vi "Smart baby safety and monitoring system.vi"() -> ()   [LabVIEW 2022 SP3]
uses:
  <vilib>/DAQmx/read.llb/DAQmx Read (Analog 1D DBL NChan 1Samp).vi
  <vilib>/DAQmx/write.llb/DAQmx Write (Digital Bool 1Line 1Point).vi
  <vilib>/DAQmx/create/channels.llb/DAQmx Create Channel (DO-Digital Output).vi
  <vilib>/DAQmx/create/channels.llb/DAQmx Create Channel (AI-Voltage-Basic).vi
  <vilib>/DAQmx/miscellaneous.llb/DAQmx Fill In Error Info.vi
panel:
  out "Cry Detected":bool
  in  "Fan Control":dbl
  in  "Vibration":tag
  out "Boolean":bool
  in  "Microphone":tag
  out "Microrphone":dbl(knob) scale=0.0..5000.0
  out "Microphone":dbl format="%0.2f"
  out "Vibration":dbl(knob) scale=-2.0..12.0
  out "Fan Speed":dbl
  out "Final":dbl
  out "Fan Activated":bool
  in  "Temp and Hum":tag
  out "Temperature":dbl(graph)
  out "Temperature":dbl(knob) scale=10.0..40.0
  out "Numeric":dbl
  out "Temperature":dbl
  out "Humidity":dbl(graph)
  out "Humidity":dbl
  out "Waveform Chart":T1(graph)
  out "Humidity":dbl(knob) scale=0.0..100.0
  in  "DAQmx Physical Channel":tag
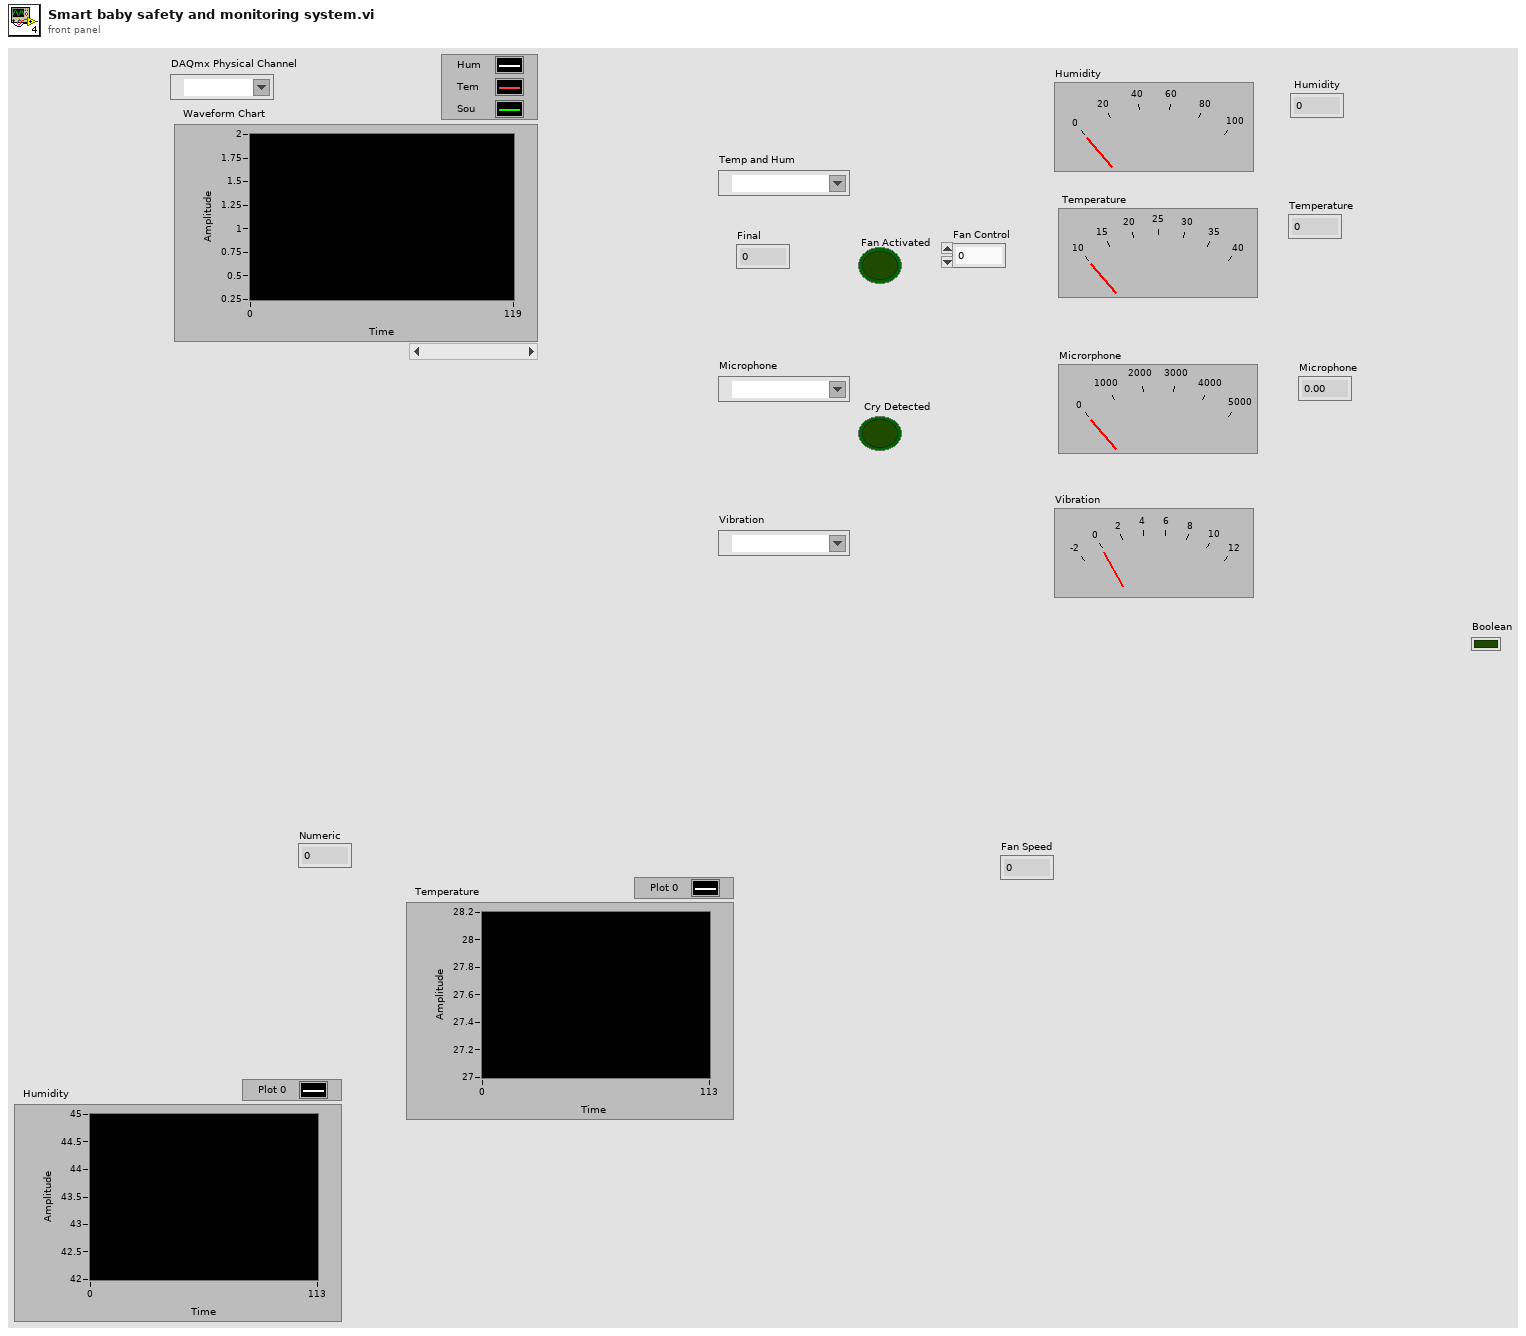
[diagram p1: front panel]
types:
  T1 = cluster{"Waveform":dbl, "Waveform":dbl, "Waveform":dbl}
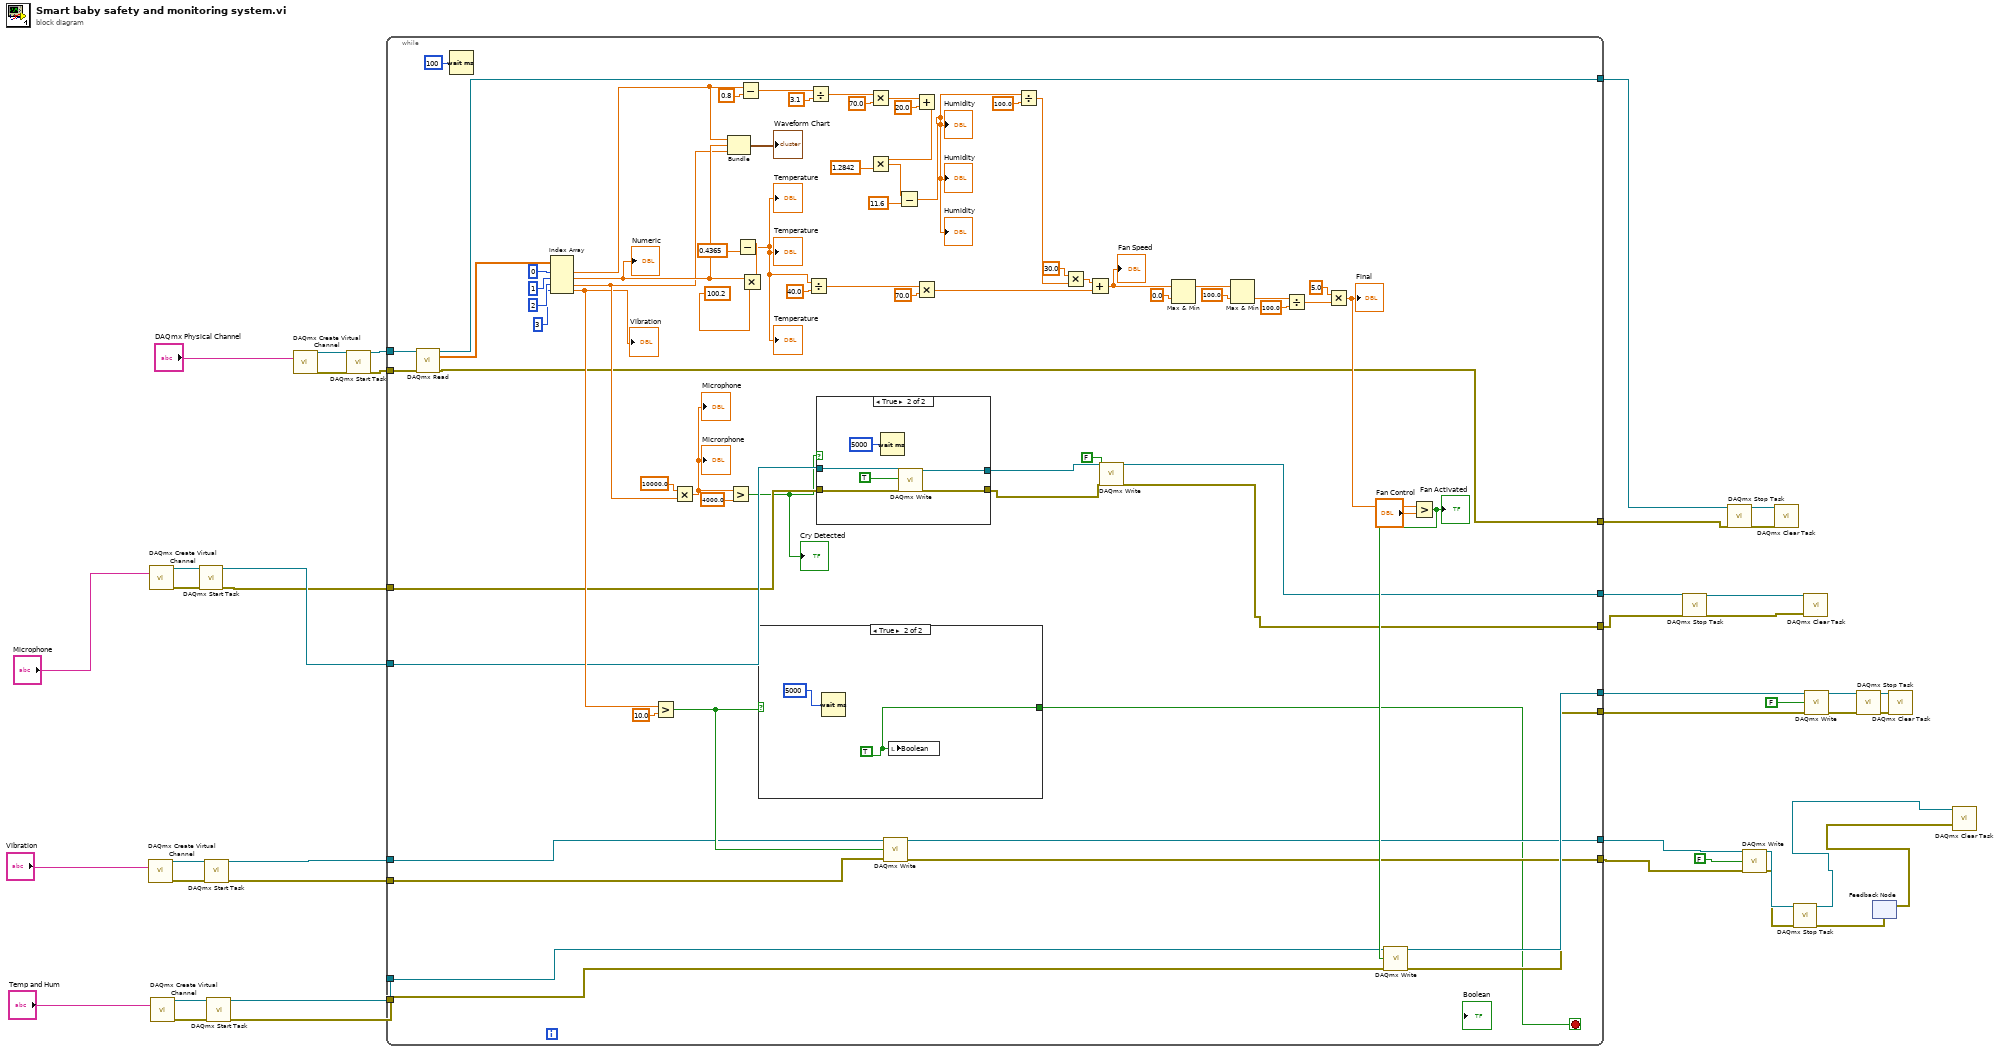
[diagram p0: block diagram]
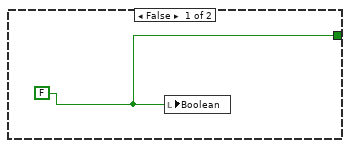
[diagram p2: hidden frame]
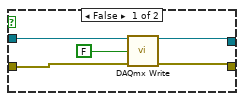
[diagram p3: hidden frame]
diagram:
  n1 = call-poly <vilib>:"DAQmx Create Virtual Channel.vi"("lines"="Vibration") -> ("task out"=w18:refnum<k21>, "error out"=w17:errorcluster)  [unwired: 13 in]
  n2 = call-poly <vilib>:"DAQmx Create Virtual Channel.vi"("lines"="Microphone") -> ("task out"=w21:refnum<k21>, "error out"=w20:errorcluster)  [unwired: 13 in]
  n3 = call-poly <vilib>:"DAQmx Create Virtual Channel.vi"("lines"="Temp and Hum") -> ("task out"=w37:refnum<k21>, "error out"=w36:errorcluster)  [unwired: 13 in]
  n4 = call <vilib>:"DAQmx Start Task.vi"("task/channels in"=w21, "error in"=w20) -> ("task out"=w19:refnum<k21>, "error out"=w4:errorcluster)  [unwired: 12 in]
  n5 = call <vilib>:"DAQmx Start Task.vi"("task/channels in"=w18, "error in"=w17) -> ("task out"=w15:refnum<k21>, "error out"=w14:errorcluster)  [unwired: 12 in]
  n6 = call <vilib>:"DAQmx Start Task.vi"("task/channels in"=w37, "error in"=w36) -> ("task out"=w24:refnum<k21>, "error out"=w23:errorcluster)  [unwired: 12 in]
  n7 = call-poly <vilib>:"DAQmx Create Virtual Channel.vi"("physical channels"="DAQmx Physical Channel") -> ("task out"=w43:refnum<k21>, "error out"=w42:errorcluster)  [unwired: 13 in]
  n8 = call <vilib>:"DAQmx Start Task.vi"("task/channels in"=w43, "error in"=w42) -> ("task out"=w39:refnum<k21>, "error out"=w38:errorcluster)  [unwired: 12 in]
  n9 = while {
    tunnel: w39 -> [w115]
    tunnel: w38 -> [w114]
    tunnel: [w65] -> w26
    tunnel: w19 -> [w56]
    tunnel: [w101] -> w33
    tunnel: [w83] -> w29
    tunnel: [w45] -> w1
    tunnel: [w46] -> w2
    tunnel: w24 -> [w64]
    tunnel: w23 -> [w63]
    tunnel: w15 -> [w54]
    tunnel: w14 -> [w53]
    tunnel: [w59] -> w9
    tunnel: [w58] -> w8
    tunnel: [w52] -> w3
    tunnel: w4 -> [w55]
    stop <- w57 stop-if-true
    n10 = call-poly <vilib>:"DAQmx Read.vi"("task/channels in"=w115, "error in"=w114) -> ("task out"=w65:refnum<k21>, "data"=w102:dbl[], "error out"=w52:errorcluster)  [unwired: 11 in]
    n11 = Wait (ms)(milliseconds to wait=u32 100) -> ()  [unwired: 1 out]
    n12 = Index Array(array=w102, index #1=0 ("index"), index #2=1 ("index"), index #3=2 ("index"), index #4=3 ("index")) -> (element #1=w85:dbl, element #2=w84:dbl, element #3=w66:dbl, element #4=w61:dbl)
    "Numeric" <- w84
    "Vibration" <- w61
    n13 = Greater?(x=w61, y=10.0) -> (0:w60:bool)
    n14 = Multiply(x=10000.0, y=w66) -> (x*y=w69:dbl)
    "Microphone" <- w69
    "Microrphone" <- w69
    n15 = Bundle("Waveform"=w85, "Waveform"=w84, "Waveform"=w66) -> (→"Waveform Chart":T1)  [unwired: 1 in]
    n16 = Greater?(x=w69, y=4000.0) -> (0:w44:bool)
    "Cry Detected" <- w44
    n17 = Subtract(x=w85, y=0.8) -> (x-y=w109:dbl)
    n18 = Multiply(x=w84, y=100.2) -> (x*y=w77:dbl)
    n19 = Subtract(x=w77, y=0.4365) -> (x-y=w76:dbl)
    "Temperature" <- w76
    "Temperature" <- w76
    "Temperature" <- w76
    n20 = case shown="True" w60 {
      tunnel: [w116 w117] -> w57
      frame False {
        w116 = FALSE
        n21 = local write "Boolean"(w116) -> ()
      }
      frame True {
        w117 = TRUE
        n22 = Wait (ms)(milliseconds to wait=u32 5000) -> ()  [unwired: 1 out]
        n23 = local write "Boolean"(w117) -> ()
      }
    }
    n24 = Divide(x=w76, y=40.0) -> (x/y=w99:dbl)
    n25 = Divide(x=w109, y=3.1) -> (x/y=w107:dbl)
    n26 = case shown="True" w44 {
      tunnel: w56 -> [w122 w128]
      tunnel: w55 -> [w121 w127]
      tunnel: [w120 w126] -> w48
      tunnel: [w119 w125] -> w47
      frame False {
        n27 = call-poly <vilib>:"DAQmx Write.vi"("task/channels in"=w122, "data"=FALSE, "error in"=w121) -> ("task out"=w120:refnum<k21>, "error out"=w119:errorcluster)  [unwired: 10 in, 1 out]
      }
      frame True {
        n28 = Wait (ms)(milliseconds to wait=u32 5000) -> ()  [unwired: 1 out]
        n29 = call-poly <vilib>:"DAQmx Write.vi"("task/channels in"=w128, "data"=TRUE, "error in"=w127) -> ("task out"=w126:refnum<k21>, "error out"=w125:errorcluster)  [unwired: 10 in, 1 out]
      }
    }
    n30 = Multiply(x=w107, y=70.0) -> (x*y=w105:dbl)
    n31 = call-poly <vilib>:"DAQmx Write.vi"("task/channels in"=w54, "data"=w60, "error in"=w53) -> ("task out"=w58:refnum<k21>, "error out"=w59:errorcluster)  [unwired: 10 in, 1 out]
    n32 = Add(x=w105, y=20.0) -> (x+y=w74:dbl)
    n33 = Multiply(x=w74, y=1.2842) -> (x*y=w72:dbl)
    n34 = Subtract(x=w72, y=11.6) -> (x-y=w71:dbl)
    "Humidity" <- w71
    "Humidity" <- w71
    "Humidity" <- w71
    n35 = Multiply(x=w99, y=70.0) -> (x*y=w93:dbl)
    n36 = Divide(x=w71, y=100.0) -> (x/y=w96:dbl)
    n37 = Multiply(x=30.0, y=w96) -> (x*y=w94:dbl)
    n38 = Add(x=w94, y=w93) -> (x+y=w80:dbl)
    "Fan Speed" <- w80
    n39 = call-poly <vilib>:"DAQmx Write.vi"("task/channels in"=w48, "data"=FALSE, "error in"=w47) -> ("task out"=w46:refnum<k21>, "error out"=w45:errorcluster)  [unwired: 10 in, 1 out]
    n40 = Max & Min(x=w80, y=0.0) -> (max(x,y)=w90:dbl)  [unwired: 1 out]
    n41 = Max & Min(x=w90, y=100.0) -> (min(x,y)=w86:dbl)  [unwired: 1 out]
    n42 = Divide(x=w86, y=100.0) -> (x/y=w88:dbl)
    n43 = Multiply(x=5.0, y=w88) -> (x*y=w82:dbl)
    "Final" <- w82
    n44 = Greater?(x=w82, y="Fan Control") -> (0:w79:bool)
    "Fan Activated" <- w79
    n45 = call-poly <vilib>:"DAQmx Write.vi"("task/channels in"=w64, "data"=w79, "error in"=w63) -> ("task out"=w101:refnum<k21>, "error out"=w83:errorcluster)  [unwired: 10 in, 1 out]
  }
  n46 = call <vilib>:"DAQmx Stop Task.vi"("task/channels in"=w2, "error in"=w1) -> ("task out"=w27:refnum<k21>, "error out"=w5:errorcluster)  [unwired: 12 in]
  n47 = call <vilib>:"DAQmx Stop Task.vi"("task/channels in"=w26, "error in"=w3) -> ("task out"=w41:refnum<k21>, "error out"=w25:errorcluster)  [unwired: 12 in]
  n48 = call-poly <vilib>:"DAQmx Write.vi"("task/channels in"=w8, "data"=FALSE, "error in"=w9) -> ("task out"=w12:refnum<k21>, "error out"=w11:errorcluster)  [unwired: 10 in, 1 out]
  n49 = call <vilib>:"DAQmx Clear Task.vi"("task in"=w41, "error in"=w25) -> ()  [unwired: 13 in, 1 out]
  n50 = call <vilib>:"DAQmx Stop Task.vi"("task/channels in"=w12, "error in"=w11) -> ("task out"=w7:refnum<k21>, "error out"=w13:errorcluster)  [unwired: 12 in]
  n51 = call <vilib>:"DAQmx Clear Task.vi"("task in"=w27, "error in"=w5) -> ()  [unwired: 13 in, 1 out]
  n52 = call-poly <vilib>:"DAQmx Write.vi"("task/channels in"=w33, "data"=FALSE, "error in"=w29) -> ("task out"=w32:refnum<k21>, "error out"=w31:errorcluster)  [unwired: 10 in, 1 out]
  n53 = call <vilib>:"DAQmx Stop Task.vi"("task/channels in"=w32, "error in"=w31) -> ("task out"=w35:refnum<k21>, "error out"=w34:errorcluster)  [unwired: 12 in]
  n54 = feedback #1() -> (w6:errorcluster)  [unwired: 1 in]
  n55 = feedback-in #1(w13) -> ()
  n56 = call <vilib>:"DAQmx Clear Task.vi"("task in"=w35, "error in"=w34) -> ()  [unwired: 13 in, 1 out]
  n57 = call <vilib>:"DAQmx Clear Task.vi"("task in"=w7, "error in"=w6) -> ()  [unwired: 13 in, 1 out]
